vi "Reply.vi"(8 "error in (no error)":errorcluster, 10 "Response":refnum<class "Message.lvclass">, 11 "Message in":refnum<class "Message.lvclass">) -> (0 "error out":errorcluster, 3 "Message out":refnum<class "Message.lvclass">)   [LabVIEW 2020, in "Stream-Simple-Msg.lvlib" / "Message.lvclass"]
uses:
  Message.lvclass
  Message.lvclass/Message.ctl
  Endpoint/Endpoint.lvclass
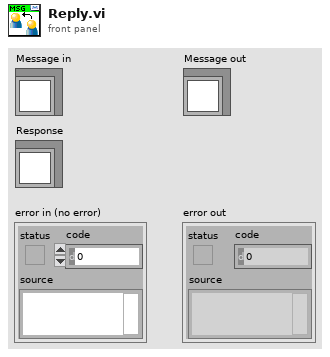
[diagram p1: front panel]
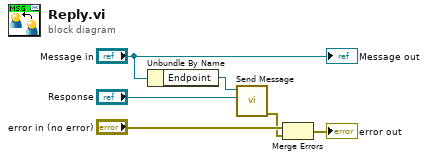
[diagram p0: block diagram]
diagram:
  n1 = Unbundle By Name("Message in") -> ("Endpoint"=w4:refnum<class "Endpoint.lvclass">)
  n2 = call "Send Message.vi"("Message"="Response", "Endpoint in"=w4) -> ("error out"=w1:errorcluster)  [unwired: 8 in, 1 out]
  n3 = Merge Errors("error in (no error)", w1) -> (→"error out":errorcluster)
  "Message out" <- "Message in"
